vi "Read MVA Coms VI Instance.vi"(8 "error in (no error)":errorcluster, 11 "MVA Comms VI in":refnum<class "MVA Comms VI Instance.lvclass">) -> (0 "error out":errorcluster, 2 "MVA Coms VI Instances":refnum<vi>, 3 "MVA Comms VI out":refnum<class "MVA Comms VI Instance.lvclass">)   [LabVIEW 2019, in "MVA Message Mapper.lvlib" / "MVA Comms VI Instance.lvclass"]
uses:
  MVA Comms VI Instance.lvclass
  MVA Comms VI Instance.lvclass/MVA Comms VI Instance.ctl
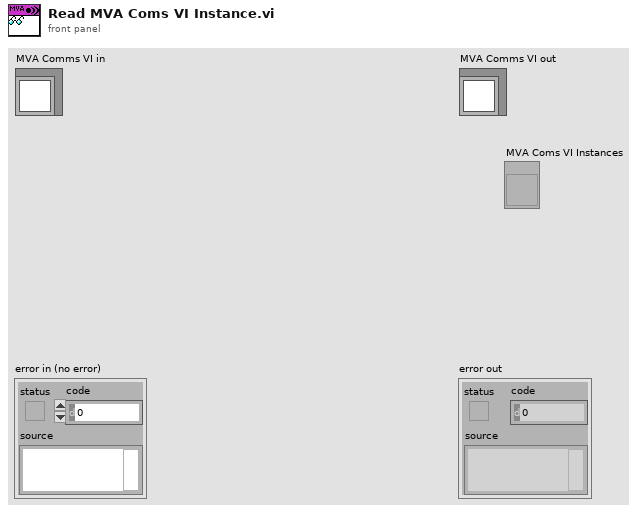
[diagram p1: front panel]
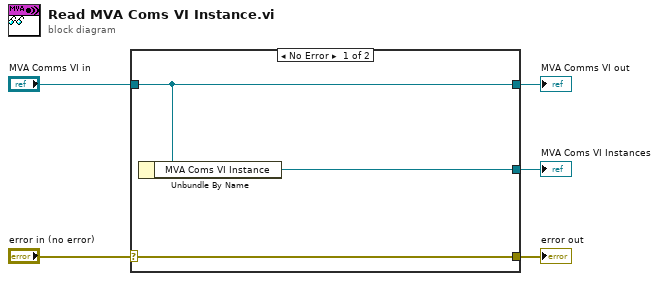
[diagram p0: block diagram]
diagram:
  n1 = case shown="No Error" "error in (no error)" {
    selector: "error in (no error)" -> [w8 w9]
    tunnel: [w8 w9] -> w4
    tunnel: [w7 w10] -> w2
    tunnel: "MVA Comms VI in" -> [w7 w10]
    tunnel: [w6 _] -> w1
    frame No Error {
      n2 = Unbundle By Name(w7) -> ("MVA Coms VI Instance"=w6:refnum<vi>)
    }
    frame Error {
    }
  }
  "error out" <- w4
  "MVA Comms VI out" <- w2
  "MVA Coms VI Instances" <- w1
